vi "Tree - Initialise.vi"(8 "error in (no error)":errorcluster, 9 "Column Headers Visible":bool, 10 "Column Header Strings[]":string[](array[string]), 11 "TreeControl in":refnum<vi>) -> (0 "error out":errorcluster, 3 "TreeControl out":refnum<vi>)   [LabVIEW 2020]
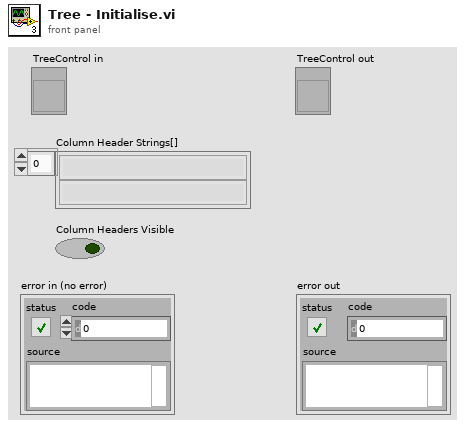
[diagram p1: front panel]
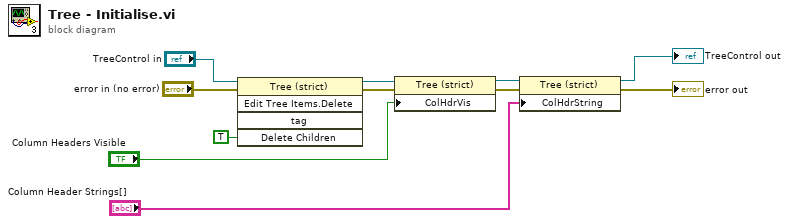
[diagram p0: block diagram]
diagram:
  n1 = invoke class="Tree (strict)" method="Edit Tree Items.Delete"(reference="TreeControl in", error in="error in (no error)", "Delete Children"=TRUE ("Delete Children?")) -> (reference out=w3:refnum<vi>, error out=w2:errorcluster)  [unwired: 2 in, 3 out]
  n2 = property class="Tree (strict)"(reference=w3, error in=w2, "ColHdrVis"="Column Headers Visible") -> (reference out=w9:refnum<vi>, error out=w10:errorcluster)
  n3 = property class="Tree (strict)"(reference=w9, error in=w10, "ColHdrString"="Column Header Strings[]") -> (reference out=→"TreeControl out":refnum<vi>, error out=→"error out":errorcluster)
